vi "SMO.Dictionary.ClearDictionary.vi"(8 "error in (no error)":errorcluster, 11 "SMO.Dictionary":refnum<class "SMO.Dictionary.lvclass">) -> (0 "error out":errorcluster, 3 "SMO.Dictionary out":refnum<class "SMO.Dictionary.lvclass">)   [LabVIEW 2013, in "SMO.Dictionary.lvlib" / "SMO.Dictionary.lvclass"]
doc: "---------------------------------------------------------------\nJKI State Machine Objects™\nhttp://jki.net/state-machine-objects/\nCopyright (C) 2005-2015, JKI <info@jki.net>\nALL RIGHTS RESERVEDJKI State Machine Objects (SMO) 1.0.0.4\nJKI - JKI\nCopyright (c) 2015, JKI"
uses:
  SMO.Dictionary.lvclass
  <vilib>/JKI/JKI SMO/SMO/SMO.lvclass
panel:
  # "For instructions on how to use the JKI State Machine Objects, examples and video tutorials, visit:\nhttp://jki.net/state-machine-objects/\n\nJKI State Machine Objects™\nhttp://jki.net/state-machine-objects/\nCopyright (C) 2005-2015, JKI <info@jki.net>\nALL RIGHTS RESERVED"
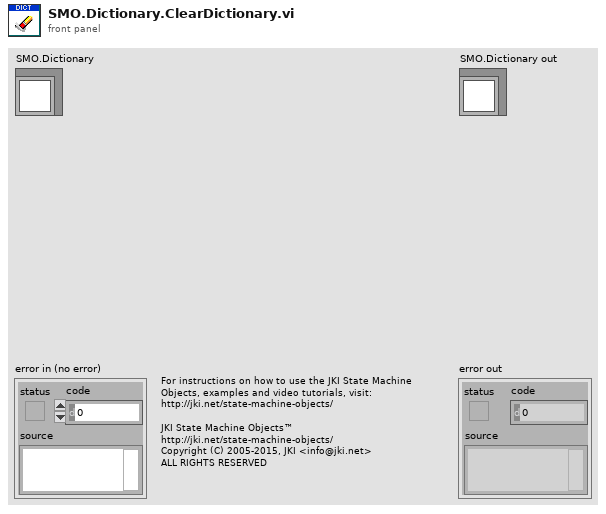
[diagram p1: front panel]
types:
  T1 = typedef "SMO.lvclass/SMOState --Enum.ctl" = enum16{"unknown", "Created", "Started", "Stopped"}
  T2 = typedef "SMO.Dictionary.lvlib/SMO.Dictionary.lvclass/PrivateEvents--Cluster.ctl" = cluster{"Update":refnum<user-event>, "Clear Dictionary":refnum<user-event>, "Delete":refnum<user-event>, "Get":refnum<user-event>, "GetMultiple":refnum<user-event>}
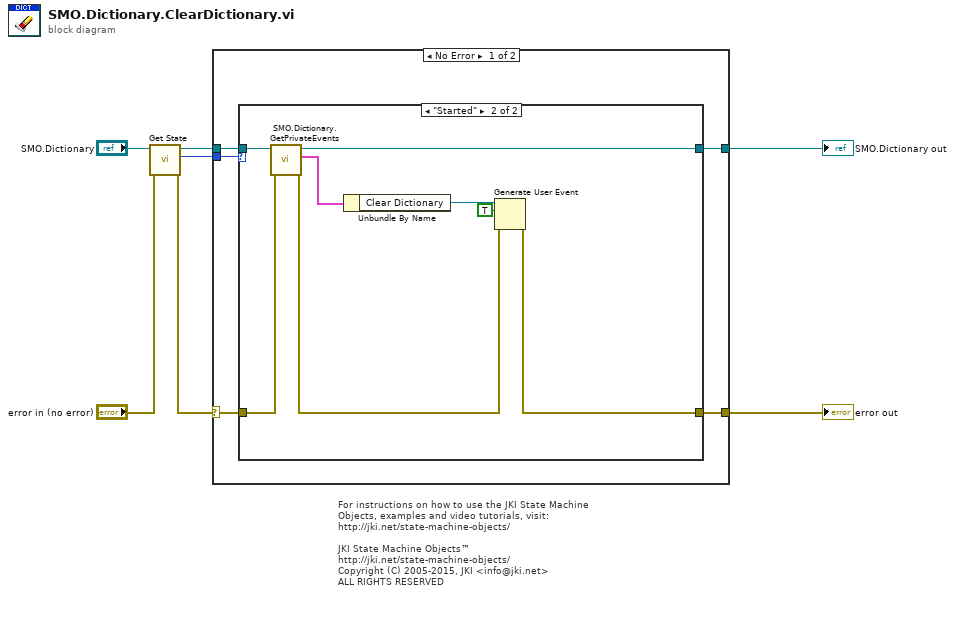
[diagram p0: block diagram]
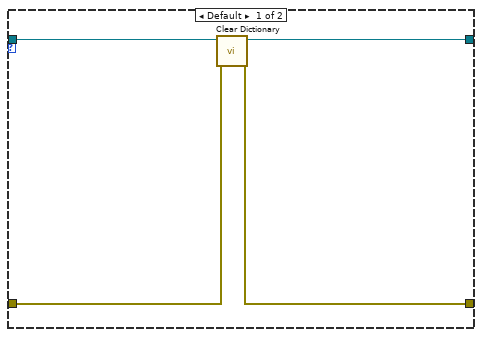
[diagram p2: hidden frame]
diagram:
  # "For instructions on how to use the JKI State Machine Objects, examples and video tutorials, visit:\nhttp://jki.net/state-machine-objects/\n\nJKI State Machine Objects™\nhttp://jki.net/state-machine-objects/\nCopyright (C) 2005-2015, JKI <info@jki.net>\nALL RIGHTS RESERVED"
  n1 = call <vilib>:"Get State.vi"("error in (no error)"="error in (no error)", "SMO"="SMO.Dictionary") -> ("error out"=w2:errorcluster, "SMO State"=w1:T1, "SMO out"=w4:refnum<class "SMO.Dictionary.lvclass">)  [unwired: 7 in]
  n2 = case shown="No Error" w2 {
    selector: w2 -> [w12 w26]
    tunnel: [w11 w26] -> w6
    tunnel: [w9 w25] -> w7
    tunnel: w4 -> [w10 w25]
    tunnel: w1 -> [w8 _]
    frame No Error {
      n3 = case shown="\"Started\"" w8 {
        tunnel: w12 -> [w14 w18]
        tunnel: [w13 w23] -> w11
        tunnel: w10 -> [w16 w20]
        tunnel: [w15 w19] -> w9
        frame Default {
          n4 = call-dynamic "Clear Dictionary.vi"("error in (no error)"=w14, "SMO.Dictionary in"=w16) -> ("error out"=w13:errorcluster, "SMO.Dictionary out"=w15:refnum<class "SMO.Dictionary.lvclass">)  [unwired: 8 in]
        }
        frame "Started" {
          n5 = call "SMO.Dictionary.GetPrivateEvents.vi"("error in (no error)"=w18, "SMO.Dictionary"=w20) -> ("error out"=w17:errorcluster, "Private Events"=w21:T2, "SMO.Dictionary out"=w19:refnum<class "SMO.Dictionary.lvclass">)  [unwired: 7 in]
          n6 = Unbundle By Name(w21) -> ("Clear Dictionary"=w24:refnum<user-event>)
          n7 = Generate User Event(user event=w24, event data cluster=TRUE ("event data"), error in=w17) -> (error out=w23:errorcluster)  [unwired: 1 in, 1 out]
        }
      }
    }
    frame Error {
    }
  }
  "error out" <- w6
  "SMO.Dictionary out" <- w7
